vi "Display_Motor_Positions.vi"(8 "error in":errorcluster={"status"=FALSE, "code"=1073676294, "source"="VISA Read in write_read.vi"}, 10 "Waypoint Number":i32, 11 "base path":path) -> (0 "error out":errorcluster={"status"=FALSE, "code"=1073676294, "source"="VISA Read in write_read.vi"}, 2 "Loaded Positions":string)   [LabVIEW 2018]
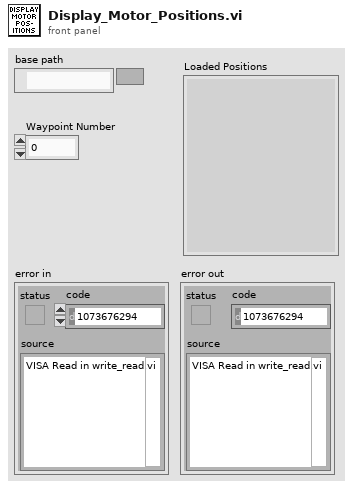
[diagram p1: front panel]
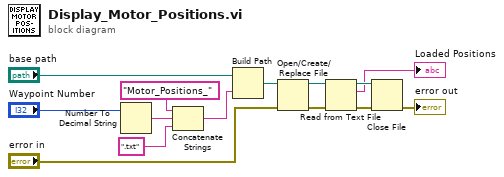
[diagram p0: block diagram]
diagram:
  n1 = Number To Decimal String(number="Waypoint Number") -> (decimal integer string=w2:string)  [unwired: 1 in]
  n2 = Concatenate Strings("Motor_Positions_" ("name or relative path"), w2, ".txt" ("name or relative path")) -> (w1:string)
  n3 = Build Path(base path="base path", name or relative path=w1) -> (appended path=w7:path)
  n4 = Open/Create/Replace File(file path (use dialog)=w7, error in="error in") -> (refnum out=w14:refnum<file>, error out=w13:errorcluster)  [unwired: 4 in, 1 out]
  n5 = Read from Text File(file (use dialog)=w14, error in=w13) -> (refnum out=w12:refnum<file>, text=→"Loaded Positions":string, error out=w11:errorcluster)  [unwired: 2 in, 1 out]
  n6 = Close File(refnum=w12, error in=w11) -> (error out=→"error out":errorcluster)  [unwired: 1 out]
